vi "ZCAN_Transmit_Queue_CAN.vi"(6 "Wait(ms)":u32, 7 "frame type":T2, 8 "error in (no error)":errorcluster caption="错误输入（无错误）", 9 "ID":u32, 10 "Datas":string, 11 "can_index_handle":u32) -> (0 "error out":errorcluster caption="错误输出", 3 "Result":bool)   [LabVIEW 2020]
uses:
  zlgcan.lvlib
  data_type/ZCAN_Transmit_Data(Queue).ctl
  bin/zlgcan_wrap.dll
  data_type/ZCANDataObj.ctl
  data_type/Agreement.ctl
  data_type/frame type.ctl
  data_type/ZCAN_TransmitFD_frame.ctl
panel:
  in  "canfd_frame":T1
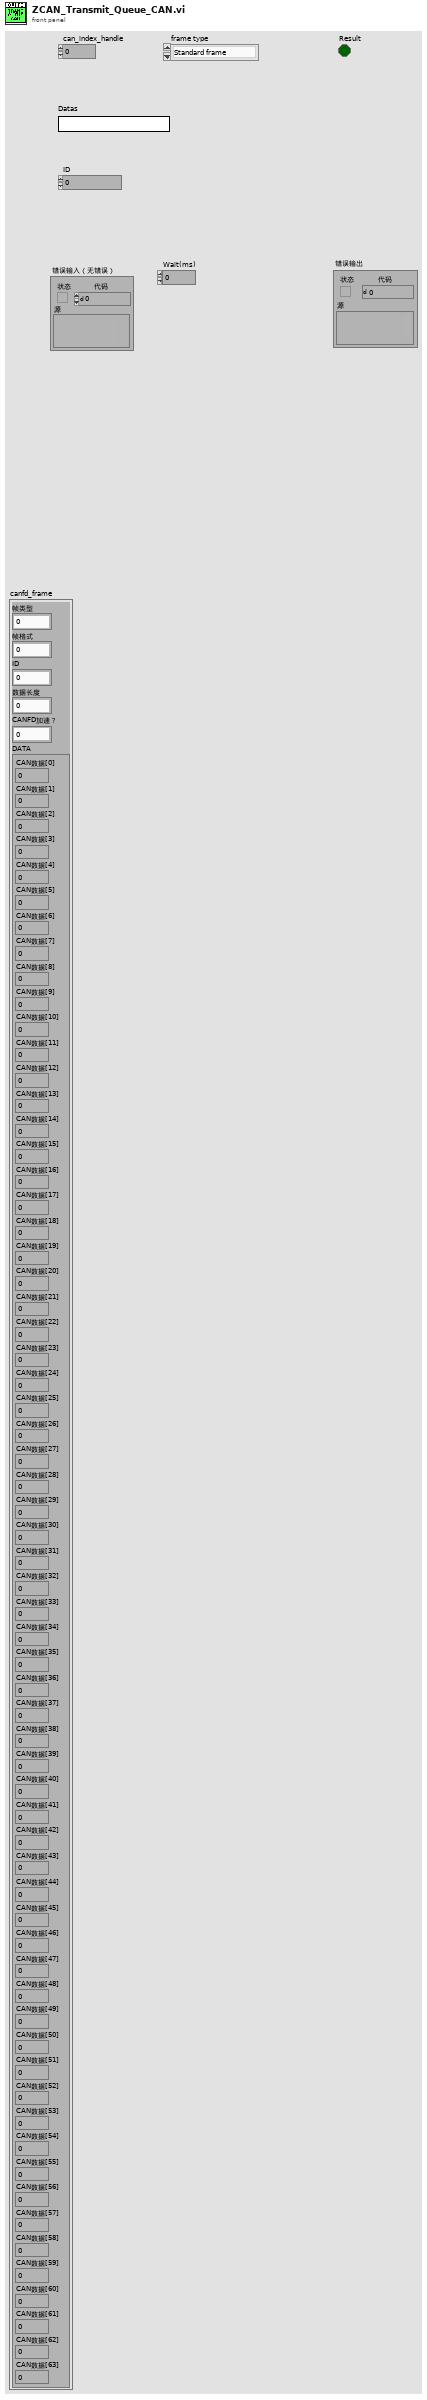
[diagram p1: front panel]
types:
  T1 = typedef "zlgcan.lvlib/ZCAN_TransmitFD_frame.ctl" = cluster{"帧类型":u32, "帧格式":u32, "ID":u32, "数据长度":u8, "CANFD加速？":u8, "DATA":cluster{"CAN数据[0]":u8, "CAN数据[1]":u8, "CAN数据[2]":u8, "CAN数据[3]":u8, "CAN数据[4]":u8, "CAN数据[5]":u8, "CAN数据[6]":u8, "CAN数据[7]":u8, "CAN数据[8]":u8, "CAN数据[9]":u8, "CAN数据[10]":u8, "CAN数据[11] ":u8, "CAN数据[12] ":u8, "CAN数据[13] ":u8, "CAN数据[14] ":u8, "CAN数据[15] ":u8, "CAN数据[16]":u8, "CAN数据[17]":u8, "CAN数据[18]":u8, "CAN数据[19]":u8, "CAN数据[20]":u8, "CAN数据[21]":u8, "CAN数据[22]":u8, "CAN数据[23]":u8, "CAN数据[24] ":u8, "CAN数据[25]":u8, "CAN数据[26]":u8, "CAN数据[27]":u8, "CAN数据[28]":u8, "CAN数据[29]":u8, "CAN数据[30]":u8, "CAN数据[31]":u8, "CAN数据[32]":u8, "CAN数据[33]":u8, "CAN数据[34]":u8, "CAN数据[35]":u8, "CAN数据[36]":u8, "CAN数据[37]":u8, "CAN数据[38]":u8, "CAN数据[39]":u8, "CAN数据[40]":u8, "CAN数据[41]":u8, "CAN数据[42]":u8, "CAN数据[43]":u8, "CAN数据[44]":u8, "CAN数据[45]":u8, "CAN数据[46]":u8, "CAN数据[47]":u8, "CAN数据[48]":u8, "CAN数据[49]":u8, "CAN数据[50]":u8, "CAN数据[51]":u8, "CAN数据[52]":u8, "CAN数据[53]":u8, "CAN数据[54]":u8, "CAN数据[55]":u8, "CAN数据[56]":u8, "CAN数据[57]":u8, "CAN数据[58]":u8, "CAN数据[59]":u8, "CAN数据[60]":u8, "CAN数据[61]":u8, "CAN数据[62]":u8, "CAN数据[63]":u8}}
  T2 = typedef "zlgcan.lvlib/frame type.ctl" = enum32{"Standard frame", "Extended frame"}
  T3 = typedef "zlgcan.lvlib/ZCAN_Transmit_Data(Queue).ctl" = cluster{"帧类型":u32, "帧格式":u32, "ID":u32, "数据长度":u8, "发送间隔":u16, "DATA":cluster{"CAN数据[0]":u8, "CAN数据[1]":u8, "CAN数据[2]":u8, "CAN数据[3]":u8, "CAN数据[4]":u8, "CAN数据[5]":u8, "CAN数据[6]":u8, "CAN数据[7]":u8}, "发送方式":u32}
  T4 = typedef "zlgcan.lvlib/Agreement.ctl" = enum16{"CAN", "CANFD"}
  T5 = typedef "zlgcan.lvlib/ZCANDataObj.ctl" = cluster{"Data_Type":u8, "CAN_CH":u8, "rawVal(未使用)":u16, "extraData[4]（未使用）":cluster{"[0]":u8, "[1]":u8, "[2]":u8, "[3]":u8}, "canCANFDData":cluster{"时间戳+混合标志位":cluster{"时间戳":u64, "混合标志位":u32}, "extraData[4]（未使用）":cluster{"[0]":u8, "[1]":u8, "[2]":u8, "[3]":u8}, "frame":cluster{"can_id":u32, "Data长度":u8, "CANFD加速？":u8, "__res0":u8, "__res1":u8, "data":cluster{"CANData[0]":u8, "CANData[1]":u8, "CANData[2]":u8, "CANData[3]":u8, "CANData[4]":u8, "CANData[5]":u8, "CANData[6]":u8, "CANData[7]":u8, "CANData[8]":u8, "CANData[9]":u8, "CANData[10]":u8, "CANData[11] ":u8, "CANData[12] ":u8, "CANData[13] ":u8, "CANData[14] ":u8, "CANData[15] ":u8, "CANData[16]":u8, "CANData[17]":u8, "CANData[18]":u8, "CANData[19]":u8, "CANData[20]":u8, "CANData[21]":u8, "CANData[22]":u8, "CANData[23]":u8, "CANData[24] ":u8, "CANData[25]":u8, "CANData[26]":u8, "CANData[27]":u8, "CANData[28]":u8, "CANData[29]":u8, "CANData[30]":u8, "CANData[31]":u8, "CANData[32]":u8, "CANData[33]":u8, "CANData[34]":u8, "CANData[35]":u8, "CANData[36]":u8, "CANData[37]":u8, "CANData[38]":u8, "CANData[39]":u8, "CANData[40]":u8, "CANData[41]":u8, "CANData[42]":u8, "CANData[43]":u8, "CANData[44]":u8, "CANData[45]":u8, "CANData[46]":u8, "CANData[47]":u8, "CANData[48]":u8, "CANData[49]":u8, "CANData[50]":u8, "CANData[51]":u8, "CANData[52]":u8, "CANData[53]":u8, "CANData[54]":u8, "CANData[55]":u8, "CANData[56]":u8, "CANData[57]":u8, "CANData[58]":u8, "CANData[59]":u8, "CANData[60]":u8, "CANData[61]":u8, "CANData[62]":u8, "CANData[63]":u8}}}, "raw":cluster{"[0]":u8, "[1]":u8, "[2]":u8, "[3]":u8, "[4]":u8, "[5]":u8, "[6]":u8, "[7]":u8, "[8]":u8, "[9]":u8, "[10]":u8, "[11]":u8, "[12]":u8, "[13]":u8, "[14]":u8, "[15]":u8, "[16]":u8, "[17]":u8, "[18]":u8, "[19]":u8, "[20]":u8, "[21]":u8, "[22]":u8, "[23]":u8, "[24]":u8, "[25]":u8, "[26]":u8, "[27]":u8, "[28]":u8, "[29]":u8, "[30]":u8, "[31]":u8, "[32]":u8, "[33]":u8, "[34]":u8, "[35]":u8, "[36]":u8, "[37]":u8, "[38]":u8, "[39]":u8, "[40]":u8, "[41]":u8, "[42]":u8, "[43]":u8, "[44]":u8, "[45]":u8, "[46]":u8, "[47]":u8, "[48]":u8, "[49]":u8, "[50]":u8, "[51]":u8, "[52]":u8, "[53]":u8, "[54]":u8, "[55]":u8, "[56]":u8, "[57]":u8, "[58]":u8, "[59]":u8, "[60]":u8, "[61]":u8, "[62]":u8, "[63]":u8, "[64]":u8, "[65]":u8, "[73]":u8, "[72]":u8, "[71]":u8, "[70]":u8, "[69]":u8, "[68]":u8, "[67]":u8, "[66]":u8, "[74]":u8, "[75]":u8, "[83]":u8, "[82]":u8, "[81]":u8, "[80]":u8, "[79]":u8, "[78]":u8, "[77]":u8, "[76]":u8, "[84]":u8, "[85]":u8, "[91]":u8, "[90]":u8, "[89]":u8, "[88]":u8, "[87]":u8, "[86]":u8}}
  T6 = cluster{"[0]":u32, "[1]":u32, "[2]":u32, "[3]":u32, "[4]":u32, "[5]":u32, "[6]":u32, "[7]":u32, "[8]":u32, "[9]":u32, "[10]":u32, "[11]":u32, "[12]":u32, "[13]":u32, "[14]":u32, "[15]":u32, "[16]":u32, "[17]":u32, "[18]":u32, "[19]":u32, "[20]":u32, "[21]":u32, "[22]":u32, "[23]":u32, "[24]":u32, "[25]":u32, "[26]":u32, "[27]":u32, "[28]":u32, "[29]":u32, "[30]":u32, "[31]":u32, "[32]":u32, "[33]":u32, "[34]":u32, "[35]":u32, "[36]":u32, "[37]":u32, "[38]":u32, "[39]":u32, "[40]":u32, "[41]":u32, "[42]":u32, "[43]":u32, "[44]":u32, "[45]":u32, "[46]":u32, "[47]":u32, "[48]":u32, "[49]":u32, "[50]":u32, "[51]":u32, "[52]":u32, "[53]":u32, "[54]":u32, "[55]":u32, "[56]":u32, "[57]":u32, "[58]":u32, "[59]":u32, "[60]":u32, "[61]":u32, "[62]":u32, "[63]":u32}
  T7 = cluster{"CANFD_data[0]":u32, "CANFD_data[1]":u32, "CANFD_data[2]":u32, "CANFD_data[3]":u32, "CANFD_data[4]":u32, "CANFD_data[5]":u32, "CANFD_data[6]":u32, "CANFD_data[7]":u32, "CANFD_data[8]":u32, "CANFD_data[9]":u32, "CANFD_data[10]":u32, "CANFD_data[11]":u32, "CANFD_data[12]":u32, "CANFD_data[13]":u32, "CANFD_data[14]":u32, "CANFD_data[15]":u32, "CANFD_data[16]":u32, "CANFD_data[17]":u32, "CANFD_data[18]":u32, "CANFD_data[19]":u32, "CANFD_data[20]":u32, "CANFD_data[21]":u32, "CANFD_data[22]":u32, "CANFD_data[23]":u32, "CANFD_data[24]":u32, "CANFD_data[25]":u32, "CANFD_data[26]":u32, "CANFD_data[27]":u32, "CANFD_data[28]":u32, "CANFD_data[29]":u32, "CANFD_data[30]":u32, "CANFD_data[31]":u32, "CANFD_data[32]":u32, "CANFD_data[33]":u32, "CANFD_data[34]":u32, "CANFD_data[35]":u32, "CANFD_data[36]":u32, "CANFD_data[37]":u32, "CANFD_data[38]":u32, "CANFD_data[39]":u32, "CANFD_data[40]":u32, "CANFD_data[41]":u32, "CANFD_data[42]":u32, "CANFD_data[43]":u32, "CANFD_data[44]":u32, "CANFD_data[45]":u32, "CANFD_data[46]":u32, "CANFD_data[47]":u32, "CANFD_data[48]":u32, "CANFD_data[49]":u32, "CANFD_data[50]":u32, "CANFD_data[51]":u32, "CANFD_data[52]":u32, "CANFD_data[53]":u32, "CANFD_data[54]":u32, "CANFD_data[55]":u32, "CANFD_data[56]":u32, "CANFD_data[57]":u32, "CANFD_data[58]":u32, "CANFD_data[59]":u32, "CANFD_data[60]":u32, "CANFD_data[61]":u32, "CANFD_data[62]":u32, "CANFD_data[63]":u32}
  T8 = cluster{cluster{"timeStamp":u64, u32}, "extraData[4]":cluster{u8, u8, u8, u8}, "canfd_frame":T1}
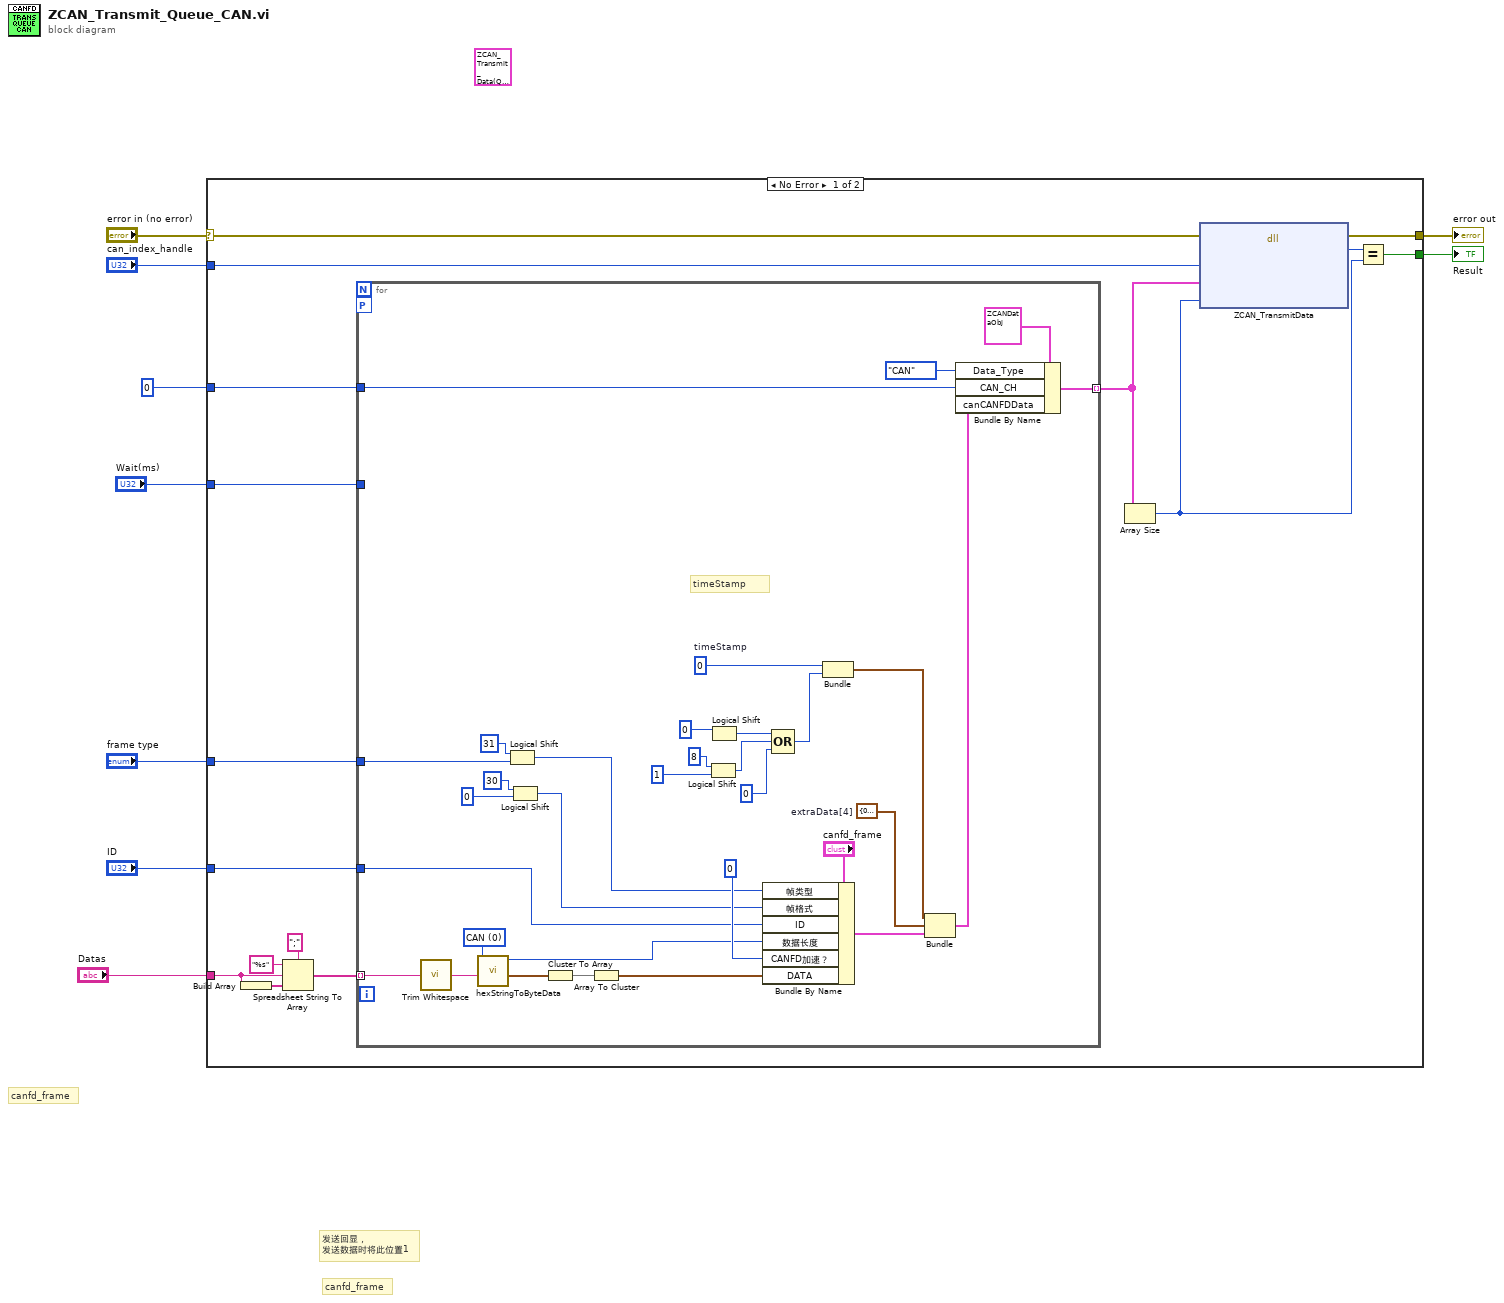
[diagram p0: block diagram]
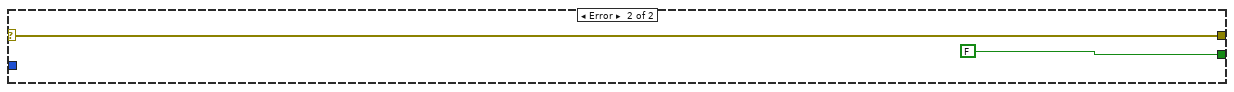
[diagram p2: hidden frame]
diagram:
  (unwired) T3 {"帧类型"=0, "帧格式"=0, "ID"=0, "数据长度"=0, "发送间隔"=0, "DATA"={"CAN数据[0]"=0, "CAN数据[1]"=0, "CAN数据[2]"=0, "CAN数据[3]"=0, "CAN数据[4]"=0, "CAN数据[5]"=0, "CAN数据[6]"=0, "CAN数据[7]"=0}, "发送方式"=0} ("ZCAN_Transmit_Data（Queue）")
  # "canfd_frame"
  # "canfd_frame"
  # "发送回显，\n发送数据时将此位置1"
  n1 = case shown="No Error" "error in (no error)" {
    selector: "error in (no error)" -> [w20 w59]
    tunnel: [w25 w59] -> w9
    tunnel: "can_index_handle" -> [w24 _]
    tunnel: "Wait(ms)" -> [w22 _]
    tunnel: "ID" -> [w21 _]
    tunnel: "Datas" -> [w14 _]
    tunnel: [w15 FALSE] -> w3
    tunnel: "frame type" -> [w13 _]
    tunnel: u8 0 ("CAN_CH") -> [w11 _]
    frame No Error {
      n2 = Build Array(w14) -> (w19:string[])
      n3 = Spreadsheet String To Array(delimiter (Tab)=";", format string="%s", spreadsheet string=w14, array type (2D Dbl)=w19) -> (array=w16:string[])
      n4 = for {
        tunnel: w22 -> [_]
        tunnel: w21 -> [w30]
        tunnel: w16 -> [w56] mode=indexing
        workers-P: _ -> [_]
        tunnel: w13 -> [w35]
        tunnel: w11 -> [w53]
        tunnel: [w36] -> w10 mode=indexing
        w42 = cluster{u8, u8, u8, u8} {0, 0, 0, 0}  # extraData[4]
        w44 = u64 0  # timeStamp
        w57 = u32 0 items=["CAN", "CANFD"] ("协议")
        # "timeStamp"
        n5 = call <vilib>:"Trim Whitespace.vi"("string"=w56) -> ("trimmed string"=w55:string)  [unwired: 1 in]
        n6 = call "hexStringToByteData.vi"("数据输入"=w55, "协议"=w57) -> ("CANFD_data"=w27:T6, "字节数"=w29:i32)  [unwired: 7 in, 1 out]
        n7 = Logical Shift(y=i16 31, x=w35) -> (x << y=w32:u32)
        n8 = Logical Shift(y=i16 30, x=i16 0) -> (x << y=w31:i16)
        n9 = Cluster To Array(cluster=w27) -> (array=w28:u32[])
        n10 = Array To Cluster(array=w28) -> (cluster=w26:T7)
        n11 = Logical Shift(y=i16 8, x=u32 1 ("y")) -> (x << y=w50:u32)
        n12 = Logical Shift(y=i16 0) -> (x << y=w49:i16)  [unwired: 1 in]
        n13 = Bundle By Name(cluster="canfd_frame", "帧类型"=w32, "帧格式"=w31, "ID"=w30, "数据长度"=w29, "CANFD加速？"=u8 0, "DATA"=w26) -> (w37:T1)
        n14 = Compound Arithmetic op=OR ("复合运算")(w49, w50, u32 0) -> (w51:u32)
        n15 = Bundle ("捆绑")("timeStamp"=w44, w51) -> (w43:cluster{"timeStamp":u64, u32})  [unwired: 1 in]
        n16 = Bundle ("捆绑")(w43, "extraData[4]"=w42, "canfd_frame"=w37) -> (w41:T8)  [unwired: 1 in]
        n17 = Bundle By Name(cluster=T5 {"Data_Type"=0, "CAN_CH"=0, "rawVal(未使用)"=0, "extraData[4]（未使用）"={"[0]"=0, "[1]"=0, "[2]"=0, "[3]"=0}, "canCANFDData"={"时间戳+混合标志位"={"时间戳"=0, "混合标志位"=0}, "extraData[4]（未使用）"={"[0]"=0, "[1]"=0, "[2]"=0, "[3]"=0}, "frame"={"can_id"=0, "Data长度"=0, "CANFD加速？"=0, "__res0"=0, "__res1"=0, "data"={"CANData[0]"=0, "CANData[1]"=0, "CANData[2]"=0, "CANData[3]"=0, "CANData[4]"=0, "CANData[5]"=0, "CANData[6]"=0, "CANData[7]"=0, "CANData[8]"=0, "CANData[9]"=0, "CANData[10]"=0, "CANData[11] "=0, "CANData[12] "=0, "CANData[13] "=0, "CANData[14] "=0, "CANData[15] "=0, "CANData[16]"=0, "CANData[17]"=0, "CANData[18]"=0, "CANData[19]"=0, "CANData[20]"=0, "CANData[21]"=0, "CANData[22]"=0, "CANData[23]"=0, "CANData[24] "=0, "CANData[25]"=0, "CANData[26]"=0, "CANData[27]"=0, "CANData[28]"=0, "CANData[29]"=0, "CANData[30]"=0, "CANData[31]"=0, "CANData[32]"=0, "CANData[33]"=0, "CANData[34]"=0, "CANData[35]"=0, "CANData[36]"=0, "CANData[37]"=0, "CANData[38]"=0, "CANData[39]"=0, "CANData[40]"=0, "CANData[41]"=0, "CANData[42]"=0, "CANData[43]"=0, "CANData[44]"=0, "CANData[45]"=0, "CANData[46]"=0, "CANData[47]"=0, "CANData[48]"=0, "CANData[49]"=0, "CANData[50]"=0, "CANData[51]"=0, "CANData[52]"=0, "CANData[53]"=0, "CANData[54]"=0, "CANData[55]"=0, "CANData[56]"=0, "CANData[57]"=0, "CANData[58]"=0, "CANData[59]"=0, "CANData[60]"=0, "CANData[61]"=0, "CANData[62]"=0, "CANData[63]"=0}}}, "raw"={"[0]"=0, "[1]"=0, "[2]"=0, "[3]"=0, "[4]"=0, "[5]"=0, "[6]"=0, "[7]"=0, "[8]"=0, "[9]"=0, "[10]"=0, "[11]"=0, "[12]"=0, "[13]"=0, "[14]"=0, "[15]"=0, "[16]"=0, "[17]"=0, "[18]"=0, "[19]"=0, "[20]"=0, "[21]"=0, "[22]"=0, "[23]"=0, "[24]"=0, "[25]"=0, "[26]"=0, "[27]"=0, "[28]"=0, "[29]"=0, "[30]"=0, "[31]"=0, "[32]"=0, "[33]"=0, "[34]"=0, "[35]"=0, "[36]"=0, "[37]"=0, "[38]"=0, "[39]"=0, "[40]"=0, "[41]"=0, "[42]"=0, "[43]"=0, "[44]"=0, "[45]"=0, "[46]"=0, "[47]"=0, "[48]"=0, "[49]"=0, "[50]"=0, "[51]"=0, "[52]"=0, "[53]"=0, "[54]"=0, "[55]"=0, "[56]"=0, "[57]"=0, "[58]"=0, "[59]"=0, "[60]"=0, "[61]"=0, "[62]"=0, "[63]"=0, "[64]"=0, "[65]"=0, "[73]"=0, "[72]"=0, "[71]"=0, "[70]"=0, "[69]"=0, "[68]"=0, "[67]"=0, "[66]"=0, "[74]"=0, "[75]"=0, "[83]"=0, "[82]"=0, "[81]"=0, "[80]"=0, "[79]"=0, "[78]"=0, "[77]"=0, "[76]"=0, "[84]"=0, "[85]"=0, "[91]"=0, "[90]"=0, "[89]"=0, "[88]"=0, "[87]"=0, "[86]"=0}} ("ZCANDataObj"), "Data_Type"=Agreement."CAN" ("Agreement"), "CAN_CH"=w53, "canCANFDData"=w41) -> (w36:T5)
      }
      n18 = Array Size(array=w10) -> (size(s)=w12:i32)
      n19 = dll-call lib="E:/Jabil tools/JabilTestLib/LV/ZLG_CANFD/bin/zlgcan_wrap.dll" fn="ZCAN_TransmitData"(error in=w20, "通道句柄"=w24, "数据帧数组"=w10, "数据帧数"=w12) -> (error out=w25:errorcluster, "返回类型"=w23:u32)  [unwired: 5 in, 1 out]
      n20 = Equal?(x=w23, y=w12) -> (x = y?=w15:bool)
    }
    frame Error {
    }
  }
  "error out" <- w9
  "Result" <- w3
